vi "Automation Timeout.vi"(8 "error in (no error)":errorcluster, 10 "Correlation ID":u32, 11 "Application in":refnum<class "Application.lvclass">) -> (0 "error out":errorcluster, 3 "Application out":refnum<class "Application.lvclass">)   [LabVIEW 2023, in "Application.lvlib" / "Application.lvclass"]
uses:
  Application.lvclass
  Application.lvclass/Application.ctl
  Automation/AutomationContext.lvclass
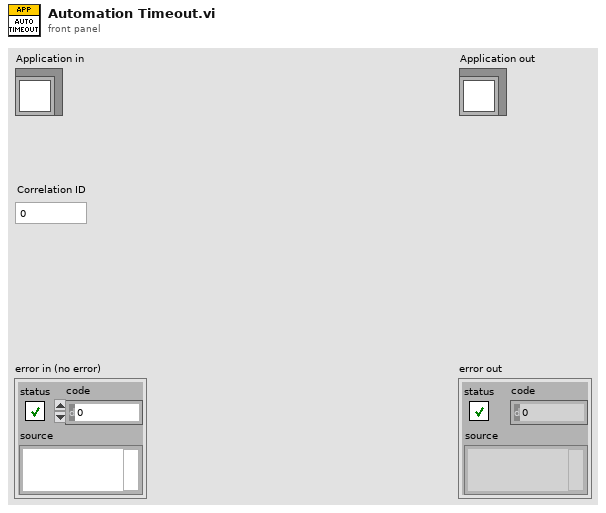
[diagram p1: front panel]
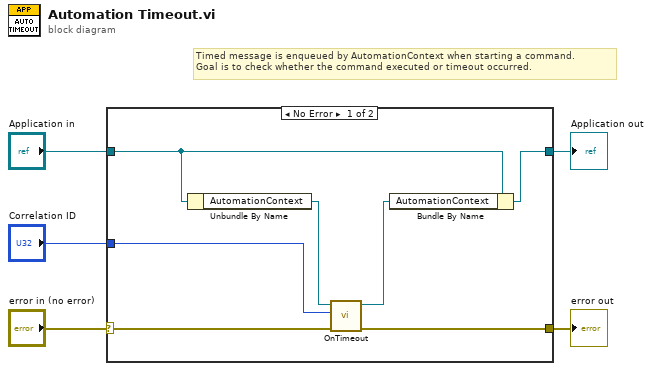
[diagram p0: block diagram]
diagram:
  # "Timed message is enqueued by AutomationContext when starting a command.\nGoal is to check whether the command executed or timeout occurred."
  n1 = case shown="No Error" "error in (no error)" {
    selector: "error in (no error)" -> [w12 w14]
    tunnel: [w11 w14] -> w4
    tunnel: [w7 w13] -> w2
    tunnel: "Application in" -> [w8 w13]
    tunnel: "Correlation ID" -> [w9 _]
    frame No Error {
      n2 = Unbundle By Name(w8) -> ("AutomationContext"=w10:refnum<class "AutomationContext.lvclass">)
      n3 = call "OnTimeout.vi"("error in (no error)"=w12, "Correlation ID"=w9, "AutomationContext in"=w10) -> ("error out"=w11:errorcluster, "AutomationContext out"=w6:refnum<class "AutomationContext.lvclass">)  [unwired: 7 in]
      n4 = Bundle By Name(cluster=w8, "AutomationContext"=w6) -> (w7:refnum<class "Application.lvclass">)
    }
    frame Error {
    }
  }
  "error out" <- w4
  "Application out" <- w2
